vi "Spin Shooter Until 14.5.vi"(9 "While Loop Runs":i32, 10 "RPM (1900)":dbl=1900.0, 11 "Execute?":bool) -> (3 "Done":bool)   [LabVIEW 2012]
uses:
  Globals/Tachometer.vi
  Globals/Motors.vi
  <vilib>/addons/control/pid/pid.llb/PID (DBL).vi
  <vilib>/addons/control/pid/NI_PID_pid.lvlib
panel:
  out "Motor Out":dbl
  in  "Shooter Wheel PID gains":T1={"proportional gain (Kc)"=0.03, "integral time (Ti, min)"=0.0, "derivative time (Td, min)"=0.0} {"derivative time (Td, min)" format="%.3f"; "integral time (Ti, min)" format="%.3f"; "proportional gain (Kc)" format="%.3f"}
  in  "Shooter Limits":cluster{"output high":dbl, "output low":dbl}={"output high"=1.0, "output low"=0.0} {"output low" format="%.2f"; "output high" format="%.2f"}
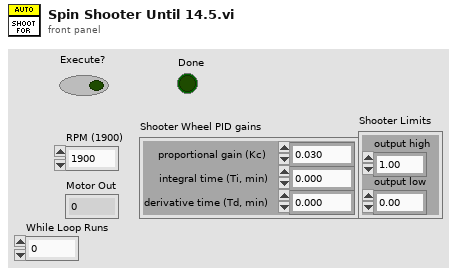
[diagram p1: front panel]
types:
  T1 = cluster{"proportional gain (Kc)":dbl, "integral time (Ti, min)":dbl, "derivative time (Td, min)":dbl}
  T2 = typedef "WPI_MotorControlDeviceRef.ctl" = cluster{"DeviceStatus":errorcluster, "Type":enum16{"PWM", "CAN"}, "PWM":cluster{"Digital Module":T3, "PWM Channel":T4, "DeadBand":T5}, "CAN":cluster{"Device Number":u8, "Control Mode":T6, "Semaphore":T7, "Max Vout":dbl}, "Invert":bool, "TransformRef":T8, "InvTransformRef":T8}
  T3 = typedef "FPGA_TypedefDigitalModule.ctl" = enum16{"Digital Module 1", "Digital Module 2"}
  T4 = typedef "FPGA_DIOPWMChannel.ctl" = enum8{"PWM 1", "PWM 2", "PWM 3", "PWM 4", "PWM 5", "PWM 6", "PWM 7", "PWM 8", "PWM 9", "PWM 10", "Invalid"}
  T5 = typedef "WPI_PWMDeadband.ctl" = cluster{"Name":string, "maxPositivePwm":i32, "minPositivePwm":i32, "centerPwm":i32, "maxNegativePwm":i32, "minNegativePwm":i32, "angularRange":u16}
  T6 = typedef "WPI_CANJaguar_ControlMode.ctl" = enum8{"Percent VBus", "Current", "Speed", "Position", "Voltage"}
  T7 = typedef "Semaphore RefNum" = refnum<k1>
  T8 = typedef "WPI_PWMTransform_ConPane.ctl" = refnum<vi>
  T9 = typedef "WPI_CounterDevRef.ctl" = cluster{"DevStatus":errorcluster, "CntIndex":T10}
  T10 = typedef "FPGA_CounterCtrSystemIndex.ctl" = enum8{"Ctr 0", "Ctr 1", "Ctr 2", "Ctr 3", "Ctr 4", "Ctr 5", "Ctr 6", "Ctr 7", "Invalid"}
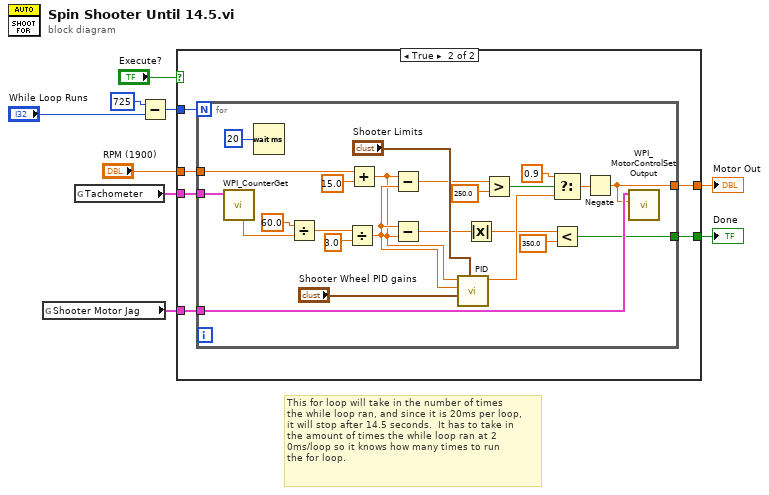
[diagram p0: block diagram]
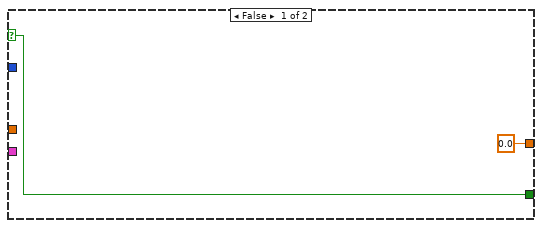
[diagram p2: hidden frame]
diagram:
  # "This for loop will take in the number of times\nthe while loop ran, and since it is 20ms per loop,\nit will stop after 14.5 seconds.  It has to take in \nthe amount of times the while loop ran at 2\n0ms/loop so it knows how many times to run \nthe for loop."
  n1 = global read "Motors.vi" "Shooter Motor Jag"() -> (w4:T2)
  n2 = global read "Tachometer.vi" "Tachometer"() -> (w6:T9)
  n3 = Subtract(x=725, y="While Loop Runs") -> (x-y=w1:i32)
  n4 = case shown="True" "Execute?" {
    selector: "Execute?" -> [w11 _]
    tunnel: [w11 w17] -> w9
    tunnel: [0.0 w16] -> w7
    tunnel: w6 -> [_ w15]
    tunnel: "RPM (1900)" -> [_ w14]
    tunnel: w4 -> [_ w13]
    tunnel: w1 -> [_ w12]
    frame False {
    }
    frame True {
      n5 = for {
        N: w12 -> [_]
        tunnel: w15 -> [w37]
        tunnel: w13 -> [w34]
        tunnel: [w22] -> w17
        tunnel: [w30] -> w16
        tunnel: w14 -> [w25]
        n6 = call <vilib>:"WPI_CounterGet.vi"("CounterDevRef in"=w37) -> ("Period (sec)"=w39:dbl)  [unwired: 5 in, 5 out]
        n7 = Wait (ms)(milliseconds to wait=u32 20) -> ()  [unwired: 1 out]
        n8 = Divide(x=60.0, y=w39) -> (x/y=w41:dbl)
        n9 = Divide(x=w41, y=3.0) -> (x/y=w24:dbl)
        n10 = Add(x=w25, y=15.0) -> (x+y=w23:dbl)
        n11 = Subtract(x=w23, y=w24) -> (x-y=w27:dbl)
        n12 = Subtract(x=w24, y=w23) -> (x-y=w20:dbl)
        n13 = call-poly <vilib>:"PID.vi"("output range"="Shooter Limits", "PID gains"="Shooter Wheel PID gains", "process variable"=w24, "setpoint"=w23) -> ("output"=w32:dbl)  [unwired: 6 in, 1 out]
        n14 = Absolute Value(x=w20) -> (abs(x)=w19:dbl)
        n15 = Greater?(x=w27, y=250.0) -> (0:w29:bool)
        n16 = Select(t=0.9, s=w29, f=w32) -> (s? t:f=w31:dbl)
        n17 = Less?(x=w19, y=350.0) -> (x < y?=w22:bool)
        n18 = Negate(x=w31) -> (-x=w30:dbl)
        n19 = call <vilib>:"WPI_MotorControlSetOutput.vi"("Output"=w30, "MotorControlDevRef"=w34) -> ()  [unwired: 7 in, 3 out]
      }
    }
  }
  "Done" <- w9
  "Motor Out" <- w7
